vi "send command.vi"(5 "Device Name":string="M1Cam") -> (2 "status":bool)   [LabVIEW 2020]
panel:
  in  "command 2":string="getMaxGUIPixel"
  out "error out":errorcluster
  out "device responds":string
  out "data out":string
  out "error message":string
  in  "command":string="getsave"
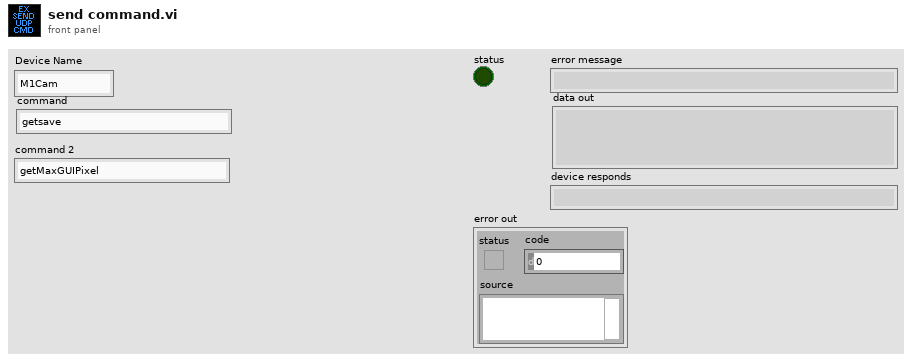
[diagram p1: front panel]
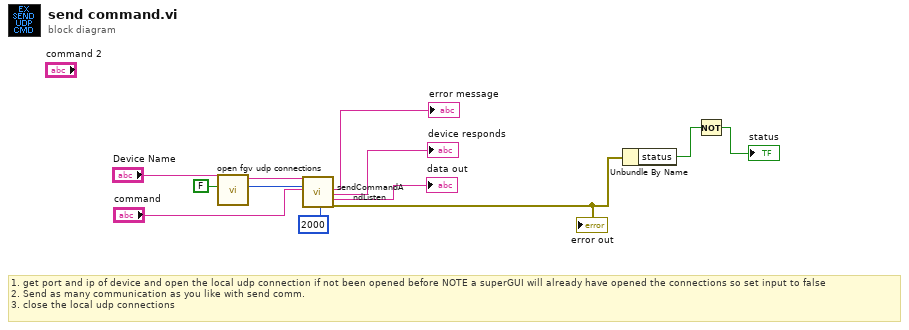
[diagram p0: block diagram]
diagram:
  # "1. get port and ip of device and open the local udp connection if not been opened before NOTE a superGUI will already have opened the connections so set input to false\n2. Send as many communication as you like with send comm.\n3. close the local udp connections"
  n1 = call "open fgv udp connections.vi"("create connection (first time only)"=FALSE, "Device Name"="Device Name") -> ("remote port"=w11:u16, "remote host ip"=w12:string)  [unwired: 8 in]
  n2 = call "sendCommandAndListen.vi"("command in"="command", "Remote Host"=w12, "port or service name"=w11, "timeout ms (100)"=2000) -> ("error message"=→"error message":string, "device responds"=→"device responds":string, "data out"=→"data out":string, "error out"=w3:errorcluster)  [unwired: 8 in, 4 out]
  "error out" <- w3
  n3 = Unbundle By Name(w3) -> ("status"=w2:bool)
  n4 = Not(x=w2) -> (.not. x?=→"status":bool)
